vi "Read (Multiple Responses).vi"(8 "error in (no error)":errorcluster, 11 "VISA resource name":refnum<visa-resource-name>) -> (0 "error out":errorcluster, 1 "Response Bundle Array":T1(array[cluster]), 2 "Response String Array":string[](array[string]), 3 "VISA resource name out":refnum<visa-resource-name>, 5 "Number of Replies":i32)   [LabVIEW 2013, in "Zaber A Series.lvlib"]
doc: "Reads all available responses from the Serial buffer within the timeout setting. An array containing the complete strings of the responses is returned on the Response String Array output, and the details of the format of the response are described here: http://www.zaber.com/wiki/Manuals/ASCII_Protocol_Manual#Replies. This VI also parses the strings, bundles the components, and returns them as an array of bundles on the Response Bundle Array pin. Additionally a pin returns the number of responses received. \n\nThis VI requires that the Initialize VI has been called with the same serial port. \n\nNote: This VI is set to a timeout of 100ms by default. This is to account for the time it may take if multiple devices are connected to complete the communication. Some commands, such as protocol changes, baud rate changes, and resetting, may take up to 500ms. Also, if fewer devices are connected this timeout could be decreased to improve lower the time this VI takes to complete."
uses:
  Zaber A Series.lvlib
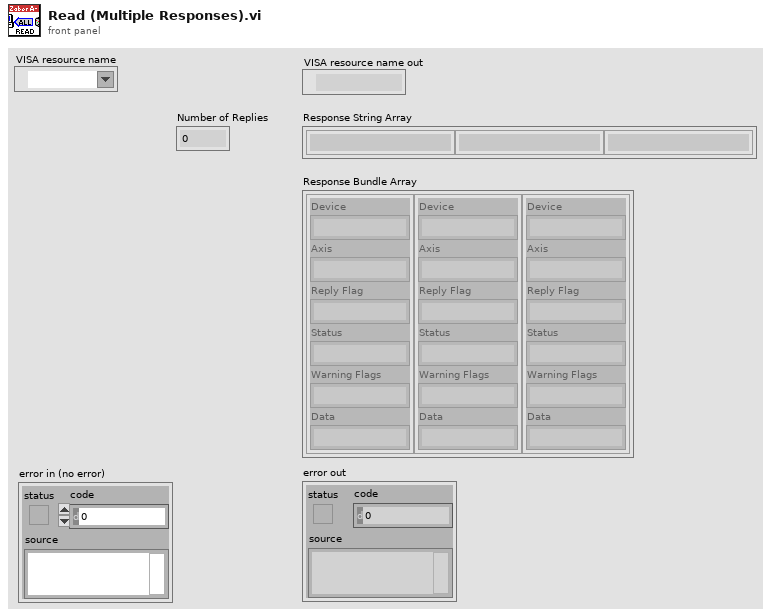
[diagram p1: front panel]
types:
  T1 = cluster{"Device":string, "Axis":string, "Reply Flag":string, "Status":string, "Warning Flags":string, "Data":string}[]
  T2 = cluster{"Device":string, "Axis":string, "Reply Flag":string, "Status":string, "Warning Flags":string, "Data":string}
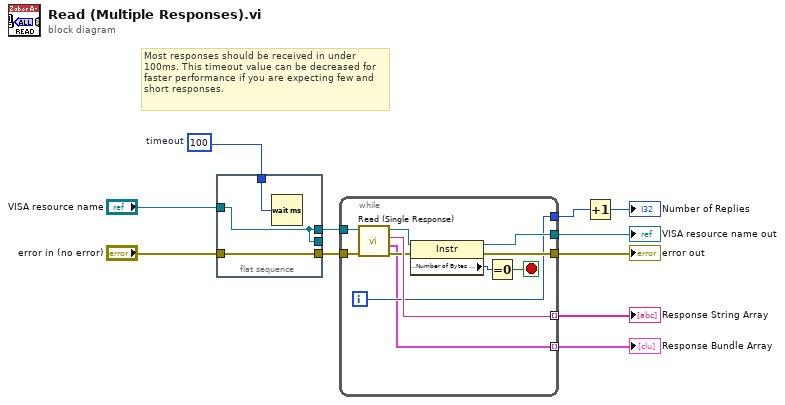
[diagram p0: block diagram]
diagram:
  w2 = u32 100  # timeout
  # "Most responses should be received in under 100ms. This timeout value can be decreased for faster performance if you are expecting few and short responses."
  n1 = flat-sequence {
    tunnel: "VISA resource name" -> [w13]
    tunnel: [w13] -> _
    tunnel: "error in (no error)" -> [w14]
    tunnel: [w14] -> w8
    tunnel: [w13] -> w9
    tunnel: w2 -> [w12]
    frame #0 {
      n2 = Wait (ms)(milliseconds to wait=w12) -> ()  [unwired: 1 out]
    }
  }
  n3 = while {
    tunnel: w9 -> [w25]
    tunnel: w8 -> [w24]
    tunnel: [w20] -> w7
    tunnel: [w21] -> w5
    tunnel: [w23] -> w6 mode=indexing
    tunnel: [w16] -> w4
    tunnel: [w15] -> w1 mode=indexing
    i -> [w16]
    stop <- w19 stop-if-true
    n4 = call "Read (Single Response).vi"("error in (no error)"=w24, "VISA resource name"=w25) -> ("error out"=w17:errorcluster, "Response Bundle"=w15:T2, "Response"=w23:string, "VISA resource name out"=w22:refnum<visa-resource-name>)  [unwired: 6 in]
    n5 = property class="Instr"(reference=w22, error in=w17) -> (reference out=w20:refnum<visa-resource-name>, error out=w21:errorcluster, "Serial Settings:Number of Bytes at Serial Port"=w18:u32)
    n6 = Equal To 0?(x=w18) -> (x = 0?=w19:bool)
  }
  "VISA resource name out" <- w7
  "error out" <- w5
  "Response String Array" <- w6
  "Response Bundle Array" <- w1
  n7 = Increment(x=w4) -> (x+1=→"Number of Replies":i32)
